vi "sutter_control2.vi"() -> ()   [LabVIEW 2016]
uses:
  <vilib>/Instr/_visa.llb/VISA Configure Serial Port (Instr).vi
panel:
  in  "下拉列表":u16(ring) items=["M1"=1, "M2"=2, "M3"=3, "M4"=4]
  in  "error in (no error)":errorcluster
  in  "Go Home":bool
  in  "stop":bool
  out "error out":errorcluster
  out "z-position":dbl
  out "y-position":dbl
  out "x-position":dbl
  in  "Z um":dbl
  in  "Y um":dbl
  in  "X um":dbl
  in  "VISA resource name":refnum<visa-resource-name>
  # "Back to (0 0 0)"
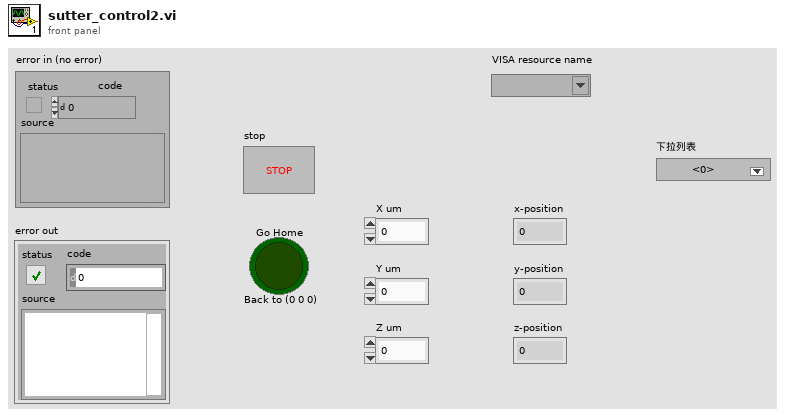
[diagram p1: front panel]
types:
  T1 = cluster{"Motor":u16, "X Pos":dbl, "Y Pos":dbl, "Z Pos":dbl, "Go Home":bool}
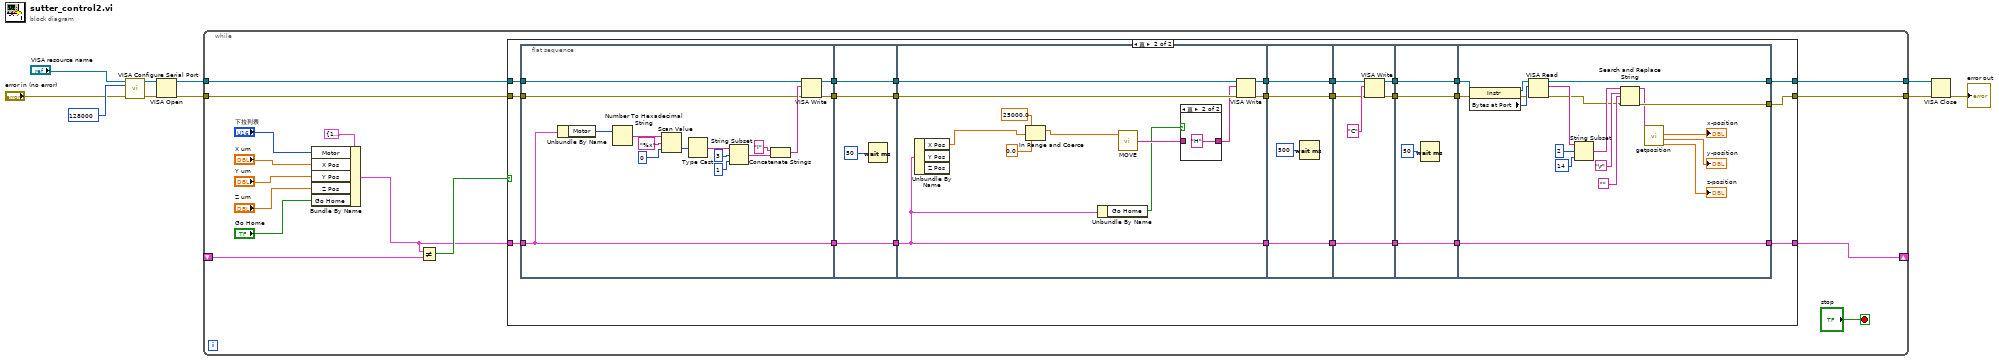
[diagram p0: block diagram]
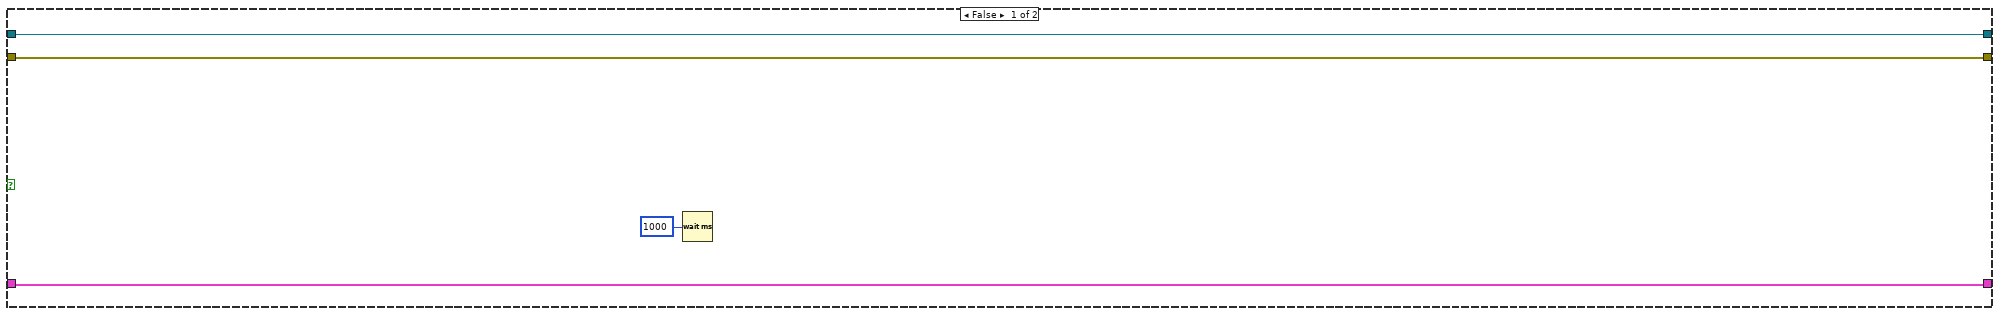
[diagram p2: hidden frame]
diagram:
  n1 = call-poly "VISA Configure Serial Port"("VISA resource name"="VISA resource name", "baud rate (9600)"=u32 128000, "error in (no error)"="error in (no error)") -> ("VISA resource name out"=w6:refnum<visa-resource-name>, "error out"=w2:errorcluster)  [unwired: 11 in]
  n2 = VISA Open(error in (no error)=w2, VISA resource name=w6) -> (VISA resource name=w5:refnum<visa-resource-name>, error out=w1:errorcluster)  [unwired: 3 in]
  n3 = while {
    tunnel: w1 -> [w22]
    tunnel: [w25] -> w7
    tunnel: w5 -> [w23]
    tunnel: [w21] -> w3
    shift-right: [w11] -> _
    shift-left: _ -> [w14]
    stop <- "stop" stop-if-true
    n4 = Bundle By Name(cluster=T1 {"Motor"=1, "X Pos"=0.0, "Y Pos"=0.0, "Z Pos"=0.0, "Go Home"=FALSE}, "Motor"="下拉列表", "X Pos"="X um", "Y Pos"="Y um", "Z Pos"="Z um", "Go Home"="Go Home") -> (w12:T1)
    n5 = Not Equal?(x=w12, y=w14) -> (x != y?=w13:bool)
    n6 = case shown="真" w13 {
      tunnel: [w26 w41] -> w25
      tunnel: w23 -> [w26 w40]
      tunnel: w22 -> [w27 w39]
      tunnel: [w27 w38] -> w21
      tunnel: w12 -> [w28 w37]
      tunnel: [w28 w30] -> w11
      frame False {
        n7 = Wait (ms)(milliseconds to wait=u32 1000 ("等待时间（毫秒）")) -> ()  [unwired: 1 out]
      }
      frame True {
        n8 = flat-sequence {
          tunnel: w39 -> [w57]
          tunnel: w40 -> [w69]
          tunnel: [w58] -> w53
          tunnel: [w56] -> w52
          tunnel: w37 -> [w54]
          tunnel: [w54] -> w31
          tunnel: [w73] -> w51
          tunnel: [w72] -> w50
          tunnel: w53 -> [w73]
          tunnel: w52 -> [w72]
          tunnel: [w70] -> w32
          tunnel: w31 -> [w70]
          tunnel: [w85] -> w49
          tunnel: [w84] -> w48
          tunnel: w51 -> [w83]
          tunnel: w50 -> [w82]
          tunnel: [w78] -> w33
          tunnel: w32 -> [w78]
          tunnel: w49 -> [w91]
          tunnel: [w91] -> w47
          tunnel: [w89] -> w46
          tunnel: w48 -> [w89]
          tunnel: [w88] -> w34
          tunnel: w33 -> [w88]
          tunnel: w47 -> [w94]
          tunnel: w46 -> [w96]
          tunnel: [w95] -> w45
          tunnel: [w93] -> w44
          tunnel: [w92] -> w35
          tunnel: w34 -> [w92]
          tunnel: w45 -> [w101]
          tunnel: [w101] -> w43
          tunnel: [w99] -> w42
          tunnel: w44 -> [w99]
          tunnel: [w98] -> w36
          tunnel: w35 -> [w98]
          tunnel: w43 -> [w115]
          tunnel: [w114] -> w41
          tunnel: w42 -> [w111]
          tunnel: [w109] -> w38
          tunnel: w36 -> [w102]
          tunnel: [w102] -> w30
          frame #0 {
            n9 = Unbundle By Name(w54) -> ("Motor"=w55:u16)
            n10 = Number To Hexadecimal String(2:w55) -> (0:w66:string)  [unwired: 1 in]
            n11 = Scan Value(string=w66, format string="%x", default (0 dbl)=0) -> (value=w64:i32)  [unwired: 1 out]
            n12 = Type Cast(x=w64) -> (*(type *) &x=w62:string)  [unwired: 1 in]
            n13 = String Subset(string=w62, offset (0)=3, length (rest)=1 ("length (rest)")) -> (substring=w59:string)
            n14 = Concatenate Strings("I" ("string"), w59) -> (w68:string)
            n15 = VISA Write(VISA resource name=w69, write buffer=w68, error in (no error)=w57) -> (VISA resource name out=w58:refnum<visa-resource-name>, error out=w56:errorcluster)  [unwired: 1 out]
          }
          frame #1 {
            n16 = Wait (ms)(milliseconds to wait=u32 50) -> ()  [unwired: 1 out]
          }
          frame #2 {
            n17 = Unbundle By Name(w78) -> ("X Pos"=w75:dbl)  [unwired: 2 out]
            n18 = In Range and Coerce ("判定范围并强制转换")(upper limit=25000.0 ("上限"), x=w75, lower limit=0.0 ("下限")) -> (coerced(x)=w74:dbl)  [unwired: 1 out]
            n19 = Unbundle By Name(w78) -> ("Go Home"=w79:bool)
            n20 = call "MOVE.vi"("x"=w74) -> ("MOVE COMMAND"=w80:string)  [unwired: 2 in]
            n21 = case shown="真" w79 {
              tunnel: [w86 "H" ("MOVE COMMAND")] -> w81
              tunnel: w80 -> [w86 _]
              frame False {
              }
              frame True {
              }
            }
            n22 = VISA Write(VISA resource name=w83, write buffer=w81, error in (no error)=w82) -> (VISA resource name out=w84:refnum<visa-resource-name>, error out=w85:errorcluster)  [unwired: 1 out]
          }
          frame #3 {
            n23 = Wait (ms)(milliseconds to wait=u32 500) -> ()  [unwired: 1 out]
          }
          frame #4 {
            n24 = VISA Write(VISA resource name=w96, write buffer="C", error in (no error)=w94) -> (VISA resource name out=w95:refnum<visa-resource-name>, error out=w93:errorcluster)  [unwired: 1 out]
          }
          frame #5 {
            n25 = Wait (ms)(milliseconds to wait=u32 50) -> ()  [unwired: 1 out]
          }
          frame #6 {
            n26 = property class="Instr"(reference=w115, error in=w111) -> (reference out=w120:refnum<visa-resource-name>, error out=w110:errorcluster, "Bytes at Port"=w116:u32)
            n27 = VISA Read(VISA resource name=w120, byte count=w116, error in (no error)=w110) -> (VISA resource name out=w114:refnum<visa-resource-name>, read buffer=w107:string, error out=w103:errorcluster)  [unwired: 1 out]
            n28 = String Subset(string=w107, offset (0)=2, length (rest)=14 ("length (rest)")) -> (substring=w104:string)
            n29 = Search and Replace String(input string=w104, search string="\r", replace string="", error in=w103) -> (result string=w108:string, error out=w109:errorcluster)  [unwired: 4 in, 2 out]
            n30 = call "getposition.vi"("string"=w108) -> ("x-position"=→"x-position":dbl, "y-position"=→"y-position":dbl, "z-position"=→"z-position":dbl)  [unwired: 1 out]
          }
        }
      }
    }
  }
  n31 = VISA Close(VISA resource name=w7, error in (no error)=w3) -> (error out=→"error out":errorcluster)
